vi "FPGA_Main.vi"() -> ()   [LabVIEW 2011]
uses:
  Battery/TypeDefs/SPI_State.ctl
  <vilib>/Platform/TimedLoop/XDataNode/timing_clust.ctl
  <vilib>/Platform/TimedLoop/XDataNode/nitl_modes.ctl
  <vilib>/Platform/TimedLoop/XDataNode/wakeup.ctl
  <vilib>/rvi/eio/common/nirviEmuTemplateMethod_errors.vi
  <vilib>/robotics/Utilities/FPGA Utilities/Generate Digital Pulse (uSec).vi
  <vilib>/Platform/TimedLoop/XDataNode/XDataNode.xnode
  <vilib>/eio/EIONode/EIONode.xnode
  <vilib>/rvi/Analysis/measure/butterworth/XNode/niFpgaButterworthFilter.xnode
  <vilib>/Platform/TimedLoop/XDataNode/XDNodeRunTimeDep.lvlib
  <vilib>/robotics/Utilities/FPGA Utilities/NI_Robotics_FPGA Utilities.lvlib
panel:
  in  "Winch Duty (uSec)":u32
  in  "Rudder Duty (uSec)":u32
  out "Battery Voltage ADC Output":u32
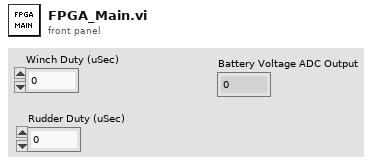
[diagram p1: front panel]
types:
  T1 = typedef "SPI_State.ctl" = enum8{"Start Read", "Transition", "Wait Cycles", "End Read"}
  T2 = typedef "XDNodeRunTimeDep.lvlib/timing_clust.ctl" = cluster{"Expected End [f-1]":u64, "Actual End [f-1]":u64, "Finished Late? [f-1]":bool, "Expected End [i-1]":u64, "Actual End [i-1]":u64, "Finished Late? [i-1]":bool, "Expected Start [i]":u64, "Actual Start [i]":u64, "Expected Start [f]":u64, "Actual Start [f]":u64, "Source Name":string, "Structure Name":string, "Period":i64, "Deadline":i64, "Offset":i64, "Start":i64, "Priority":i32, "Timeout":i32, "Mode":T3, "Wakeup Reason":T4, "Error":errorcluster, "Source Type":string, "Secondary Source Type":string, "Global End Time":u64, "Global Start Time":u64, "Frame Duration":u64, "Iteration Duration":u64, "Assigned CPU":i32, "I/O Scan Engine Mode":u32}
  T3 = typedef "XDNodeRunTimeDep.lvlib/nitl_modes.ctl" = enum32{"No Change", "Process missed periods, maintain original phase", "Discard missed periods, maintain original phase", "Process missed periods, ignore original phase", "Discard missed periods, ignore original phase"}
  T4 = typedef "XDNodeRunTimeDep.lvlib/wakeup.ctl" = enum32{"Normal", "Aborted", "Asynchronous wakeup", "Timing source error", "Timed loop error", "Timeout"}
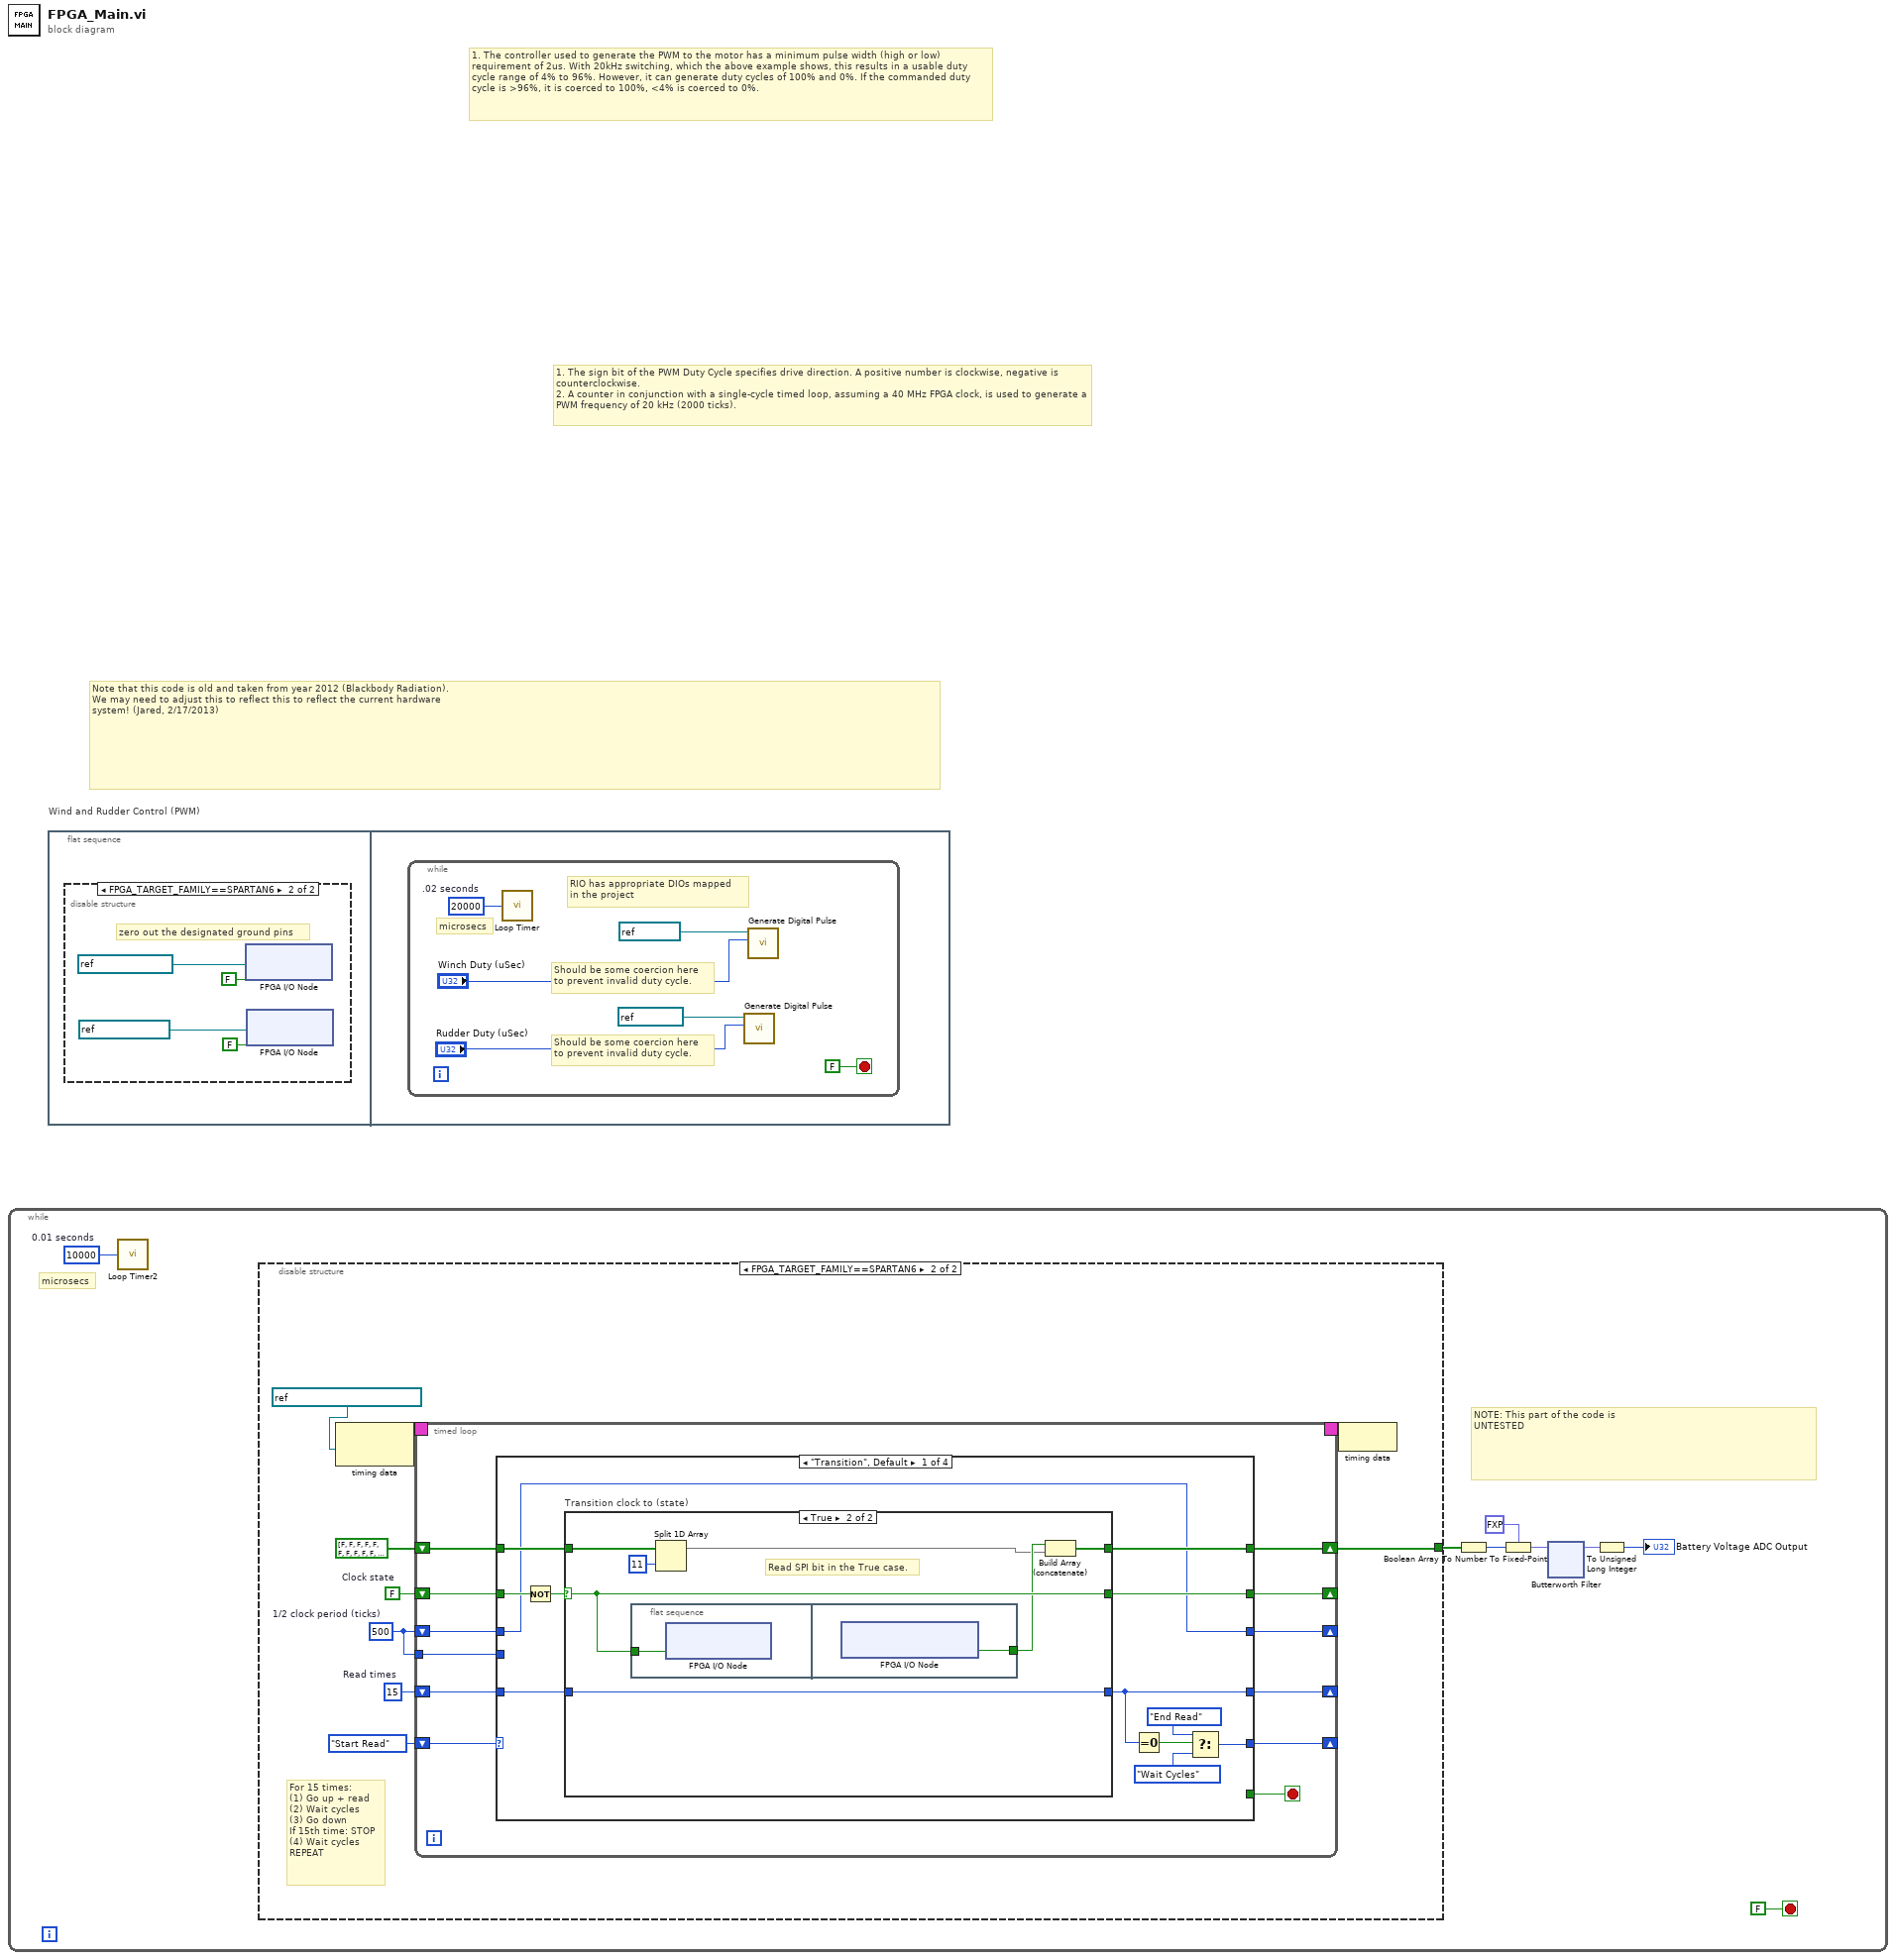
[diagram p0: block diagram]
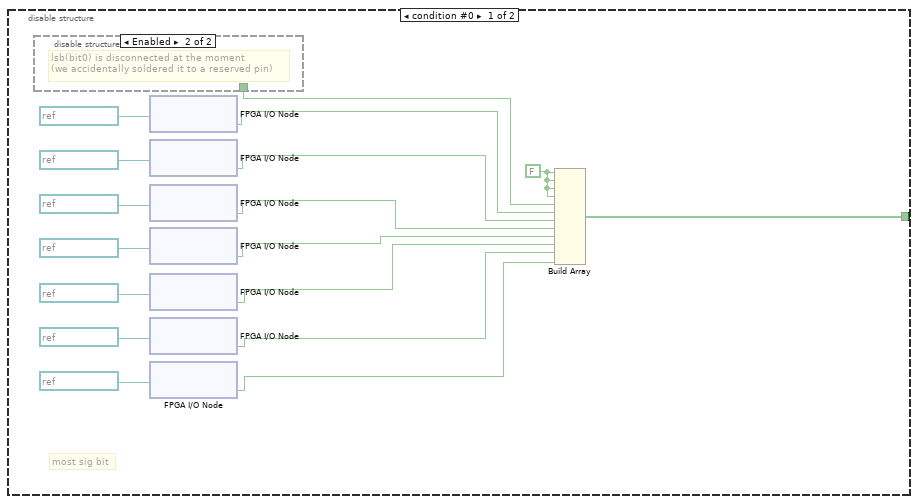
[diagram p3: hidden frame]
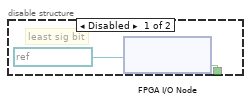
[diagram p4: hidden frame]
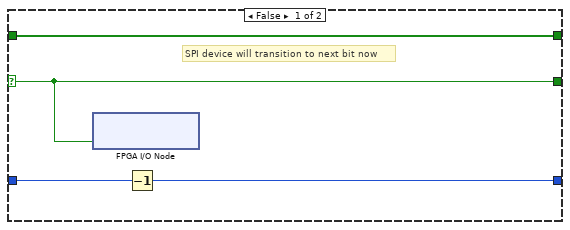
[diagram p5: hidden frame]
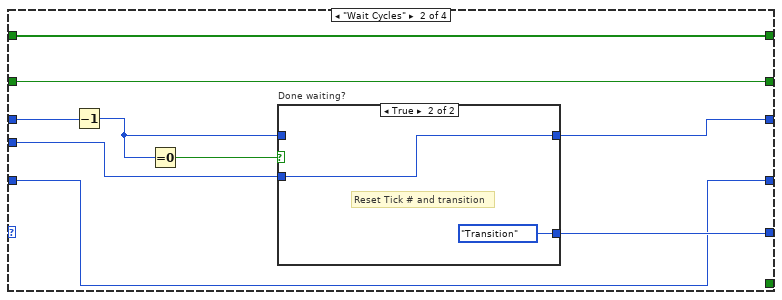
[diagram p6: hidden frame]
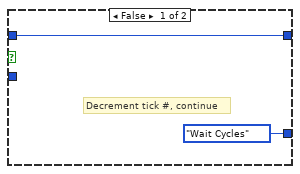
[diagram p7: hidden frame]
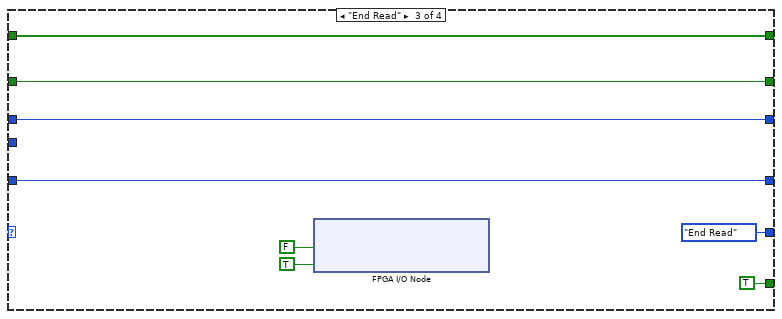
[diagram p8: hidden frame]
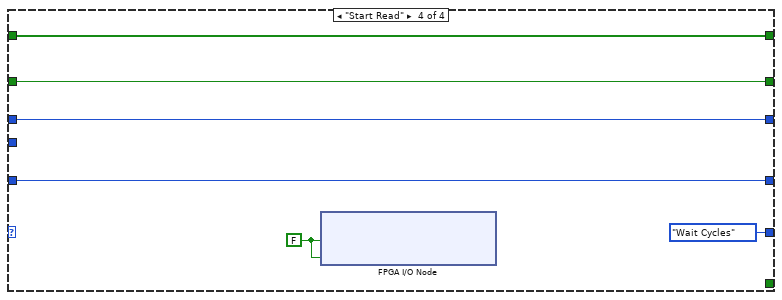
[diagram p9: hidden frame]
diagram:
  # "Note that this code is old and taken from year 2012 (Blackbody Radiation).\nWe may need to adjust this to reflect this to reflect the current hardware\nsystem! (Jared, 2/17/2013)"
  # "1. The sign bit of the PWM Duty Cycle specifies drive direction. A positive number is clockwise, negative is counterclockwise.\n2. A counter in conjunction with a single-cycle timed loop, assuming a 40 MHz FPGA clock, is used to generate a PWM frequency of 20 kHz (2000 ticks)."
  # "1. The controller used to generate the PWM to the motor has a minimum pulse width (high or low) requirement of 2us. With 20kHz switching, which the above example shows, this results in a usable duty cycle range of 4% to 96%. However, it can generate duty cycles of 100% and 0%. If the commanded duty cycle is >96%, it is coerced to 100%, <4% is coerced to 0%."
  n1 = while {
    stop <- FALSE stop-if-true
    w1 = u32 10000  # 0.01 seconds
    # "microsecs"
    # "NOTE: This part of the code is\nUNTESTED"
    n2 = call "Loop Timer2"("Count(uSec)"=w1) -> ()  [unwired: 1 out]
    n3 = disable-structure shown="FPGA_TARGET_FAMILY==SPARTAN6" {
      disable-tunnel: [w18 w39] -> w8
      frame condition #0 {
        w17 = FALSE ("element")
        # "most sig bit"
        n4 = disable-structure shown="Enabled" {
          disable-tunnel: [w34 _] -> w19
          frame Disabled {
            # "least sig bit"
            n5 = xnode "FPGA I/O Node"("FPGA I/O In"=refnum<k21> "VBatt bit0") -> ("I/O Item"=w34:bool)  [unwired: 1 out]
          }
          frame Enabled {
            # "lsb(bit0) is disconnected at the moment\n(we accidentally soldered it to a reserved pin)"
          }
        }
        n6 = xnode "FPGA I/O Node"("FPGA I/O In"=refnum<k21> "VBatt bit1") -> ("I/O Item"=w27:bool)  [unwired: 1 out]
        n7 = xnode "FPGA I/O Node"("FPGA I/O In"=refnum<k21> "VBatt bit2") -> ("I/O Item"=w28:bool)  [unwired: 1 out]
        n8 = xnode "FPGA I/O Node"("FPGA I/O In"=refnum<k21> "VBatt bit3") -> ("I/O Item"=w29:bool)  [unwired: 1 out]
        n9 = xnode "FPGA I/O Node"("FPGA I/O In"=refnum<k21> "VBatt bit4") -> ("I/O Item"=w30:bool)  [unwired: 1 out]
        n10 = xnode "FPGA I/O Node"("FPGA I/O In"=refnum<k21> "VBatt bit5") -> ("I/O Item"=w31:bool)  [unwired: 1 out]
        n11 = xnode "FPGA I/O Node"("FPGA I/O In"=refnum<k21> "VBatt bit6") -> ("I/O Item"=w32:bool)  [unwired: 1 out]
        n12 = xnode "FPGA I/O Node"("FPGA I/O In"=refnum<k21> "VBatt bit7") -> ("I/O Item"=w33:bool)  [unwired: 1 out]
        n13 = Build Array(w17, w17, w17, w17, w19, w27, w28, w29, w30, w31, w32, w33) -> (w18:bool[])
      }
      frame condition #1 (active) {
        w40 = u32 500  # 1/2 clock period (ticks)
        w41 = FALSE  # Clock state
        w42 = u8 15  # Read times
        # "For 15 times:\n(1) Go up + read\n(2) Wait cycles\n(3) Go down\nIf 15th time: STOP\n(4) Wait cycles\nREPEAT"
        n14 = node-c288(refnum<k21> "40 MHz Onboard Clock" ("Source Name")) -> (w38:T2)
        n15 = timed-loop {
          shift-right: [w49] -> _
          shift-left: SPI_State."Start Read" ("Action") -> [w56]
          shift-right: [w52] -> w39
          shift-left: bool[] [FALSE, FALSE, FALSE, FALSE, FALSE, FALSE, FALSE, FALSE, FALSE, FALSE, FALSE, FALSE] ("Battery Voltage") -> [w53]
          shift-right: [w54] -> _
          shift-left: w41 -> [w55]
          tunnel: w40 -> [w47]
          shift-right: [w46] -> _
          shift-left: w40 -> [w48]
          shift-right: [w50] -> _
          shift-left: w42 -> [w51]
          timing: w38 -> [_]
          timing-out: [_] -> w37
          stop <- w45 stop-if-true
          n16 = case shown="\"Transition\", Default" w56 {
            tunnel: w55 -> [w68 w90 w98 w106]
            tunnel: [w67 w90 w98 w106] -> w54
            tunnel: w53 -> [w65 w89 w97 w107]
            tunnel: [w64 w89 w97 w107] -> w52
            tunnel: w51 -> [w63 w82 w101 w104]
            tunnel: [w61 w82 w101 w104] -> w50
            tunnel: [w59 w85 SPI_State."End Read" ("Action") SPI_State."Wait Cycles" ("Action")] -> w49
            tunnel: w48 -> [w62 w88 w99 w105]
            tunnel: w47 -> [_ w83 _ _]
            tunnel: [w62 w84 w99 w105] -> w46
            tunnel: [_ _ TRUE _] -> w45
            frame "Transition", Default {
              n17 = Not(x=w68) -> (.not. x?=w66:bool)
              n18 = case "Transition clock to (state)" shown="True" w66 {
                selector: w66 -> [w72 w79]
                tunnel: [w72 w79] -> w67
                tunnel: w65 -> [w69 w75]
                tunnel: [w69 w73] -> w64
                tunnel: w63 -> [w71 w77]
                tunnel: [w70 w77] -> w61
                frame False {
                  # "SPI device will transition to next bit now"
                  n19 = xnode "FPGA I/O Node"("VBatt_Clock"=w72) -> ()  [unwired: 1 in, 1 out]
                  n20 = Decrement(x=w71) -> (x-1=w70:u8)
                }
                frame True {
                  # "Read SPI bit in the True case."
                  n21 = flat-sequence {
                    tunnel: w79 -> [w80]
                    tunnel: [w81] -> w76
                    frame #0 {
                      n22 = xnode "FPGA I/O Node"("VBatt_Clock"=w80) -> ()  [unwired: 1 in, 1 out]
                    }
                    frame #1 {
                      n23 = xnode "FPGA I/O Node"() -> ("VBatt_DigitalInput"=w81:bool)  [unwired: 1 in, 1 out]
                    }
                  }
                  n24 = Split 1D Array(array=w75, index=11) -> (first subarray=w74:bool[])  [unwired: 1 out]
                  n25 = Build Array (concatenate)(w76, w74) -> (w73:bool[])
                }
              }
              n26 = Equal To 0?(x=w61) -> (x = 0?=w60:bool)
              n27 = Select(t=SPI_State."End Read" ("Action"), s=w60, f=SPI_State."Wait Cycles" ("Action")) -> (s? t:f=w59:T1)
            }
            frame "Wait Cycles" {
              n28 = Decrement(x=w88) -> (x-1=w86:u32)
              n29 = Equal To 0?(x=w86) -> (x = 0?=w87:bool)
              n30 = case "Done waiting?" shown="True" w87 {
                tunnel: w86 -> [w91 _]
                tunnel: [SPI_State."Wait Cycles" ("Action") SPI_State."Transition" ("Action")] -> w85
                tunnel: [w91 w93] -> w84
                tunnel: w83 -> [_ w93]
                frame False {
                  # "Decrement tick #, continue"
                }
                frame True {
                  # "Reset Tick # and transition"
                }
              }
            }
            frame "End Read" {
              n31 = xnode "FPGA I/O Node"("VBatt_Clock"=FALSE ("VBatt_ChipSelectInverted"), "VBatt_ChipSelectInverted"=TRUE) -> ()  [unwired: 2 in, 2 out]
            }
            frame "Start Read" {
              w108 = FALSE ("VBatt_ChipSelectInverted")
              n32 = xnode "FPGA I/O Node"("VBatt_Clock"=w108, "VBatt_ChipSelectInverted"=w108) -> ()  [unwired: 2 in, 2 out]
            }
          }
        }
        n33 = node-c288(w37) -> ()
      }
    }
    n34 = Boolean Array To Number(Boolean array=w8) -> (number=w7:u16)
    n35 = To Fixed-Point(fixed-point type=fxp<+/-,32,33> 0.0 ("input data"), number=w7) -> (fixed-point=w5:fxp<+/-,32,33>)
    n36 = xnode "Butterworth Filter"("input data"=w5) -> ("output data"=w4:fxp<+/-,32,33>)  [unwired: 2 in]
    n37 = To Unsigned Long Integer(number=w4) -> (unsigned 32bit integer=→"Battery Voltage ADC Output":u32)
  }
  n38 = flat-sequence "Wind and Rudder Control (PWM)" {
    frame #0 {
      n39 = disable-structure shown="FPGA_TARGET_FAMILY==SPARTAN6" {
        frame condition #0 {
        }
        frame condition #1 (active) {
          # "zero out the designated ground pins"
          n40 = xnode "FPGA I/O Node"("I/O Item"=FALSE, "FPGA I/O In"=refnum<k21> "Rudder_GND" ("FPGA digital output")) -> ()  [unwired: 1 out]
          n41 = xnode "FPGA I/O Node"("I/O Item"=FALSE, "FPGA I/O In"=refnum<k21> "Winch_GND" ("FPGA digital output")) -> ()  [unwired: 1 out]
        }
      }
    }
    frame #1 {
      n42 = while {
        stop <- FALSE stop-if-true
        w122 = u32 20000  # .02 seconds
        # "microsecs"
        # "Should be some coercion here\nto prevent invalid duty cycle."
        # "Should be some coercion here\nto prevent invalid duty cycle."
        # "RIO has appropriate DIOs mapped\nin the project"
        n43 = call "Loop Timer"("Count(uSec)"=w122) -> ()  [unwired: 1 out]
        n44 = call-poly <vilib>:"Generate Digital Pulse.vi"("pulse width (uSec)"="Rudder Duty (uSec)", "FPGA digital output"=refnum<k21> "Rudder") -> ()  [unwired: 10 in]
        n45 = call-poly <vilib>:"Generate Digital Pulse.vi"("pulse width (uSec)"="Winch Duty (uSec)", "FPGA digital output"=refnum<k21> "Winch") -> ()  [unwired: 10 in]
      }
    }
  }
